vi "Change Tag Name.vi"(6 "Variant":variant, 8 "error in":errorcluster, 9 "old values":string[][](array[string]), 10 "object ref in":T1, 11 "Cluster":T2) -> (0 "error out":errorcluster)   [LabVIEW 2013, in "Shared Memory Editor Node.lvclass"]
doc: "Copyright 2016 National Instruments Corporation\n\nLicensed under the Apache License, Version 2.0 (the \"License\"); you may not use this file except in compliance with the License. You may obtain a copy of the License at http://www.apache.org/licenses/LICENSE-2.0\nUnless required by applicable law or agreed to in writing, software distributed under the License is distributed on an \"AS IS\" BASIS, WITHOUT WARRANTIES OR CONDITIONS OF ANY KIND, either express or implied. See the License for the specific language governing permissions and limitations under the License."
uses:
  Shared Memory Editor Node.lvclass
  <vilib>/NI/DCAF Table API/Table Manager/Cell Change.ctl
  <vilib>/NI/DCAF Table API/Table Manager/object ref.ctl
  <vilib>/NI/DCAF/Tag Editor Core/Configuration Editor/Classes/Engine Parent/Engine Parent Editor Node.lvclass
  <vilib>/NI/DCAF/Tag Editor Core/Configuration Editor/Classes/Module editor node/module editor node.lvclass
  module/configuration/Shared Memory Configuration.lvclass
  module/configuration/Shared Memory Configuration.lvclass/Shared Memory Configuration.ctl
  <vilib>/NI/DCAF Table API/Table Manager.lvlib
  <vilib>/NI/DCAF Table API/Table Manager/Table Manager.lvclass
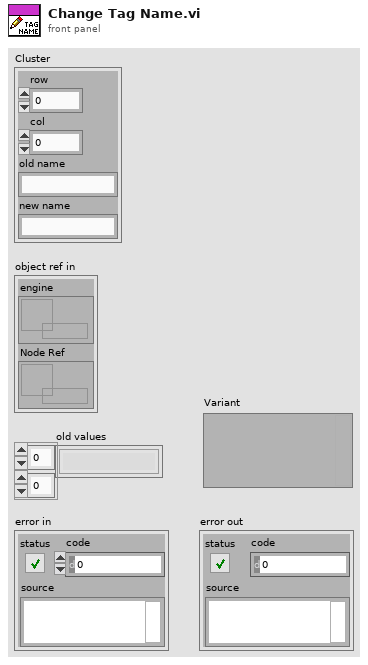
[diagram p1: front panel]
types:
  T1 = typedef "Table Manager.lvlib/Table Manager.lvclass/object ref.ctl" = cluster{"engine":refnum<data-value>, "Node Ref":refnum<data-value>}
  T2 = typedef "Table Manager.lvlib/Cell Change.ctl" = cluster{"row":i32, "col":i32, "old name":string, "new name":string}
  T3 = typedef "Shared Memory Configuration.lvclass/line configuration.ctl" = cluster{"name":string, "data type":T4, "channel":refnum<class "TBM channel.lvclass">}
  T4 = typedef "tag bus.lvlib/tag descriptor.lvclass/Data Type.ctl" = enum16{"Double", "Single", "I64", "I32", "I16", "I8", "U64", "U32", "U16", "U8", "Boolean", "String", "Array of Double", "Array of Single", "Array of I64", "Array of I32", "Array of I16", "Array of I8", "Array of U64", "Array of U32", "Array of U16", "Array of U8", "Array of Boolean", "Array of String"}
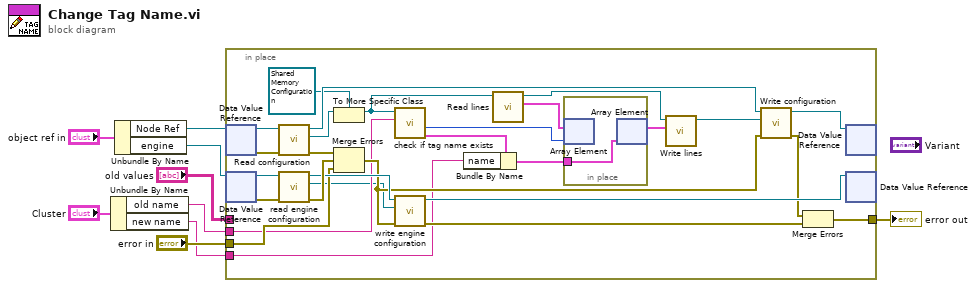
[diagram p0: block diagram]
diagram:
  n1 = Unbundle By Name("Cluster") -> ("old name"=w2:string, "new name"=w1:string)
  n2 = Unbundle By Name("object ref in") -> ("Node Ref"=w4:refnum<data-value>, "engine"=w3:refnum<data-value>)
  n3 = in-place {
    in-place-border: [w29] -> w8
    in-place-border: "error in" -> [w21]
    in-place-border: "old values" -> [_]
    in-place-border: w2 -> [w15]
    in-place-border: w1 -> [w11]
    n4 = in-place-dvr #1(w4) -> (w26:refnum<class "module editor node.lvclass">, w28:errorcluster)
    n5 = in-place-dvr #2(w3) -> (w36:refnum<class "Engine Parent Editor Node.lvclass">, w37:errorcluster)
    n6 = call-dynamic "Read configuration.vi"("error in"=w28, "NISE_CEF_serializable node in"=w26) -> ("error out"=w27:errorcluster, "configuration"=w24:refnum<class "NISE_CEF_serializable configuration.lvclass">, "NISE_CEF_serializable node out"=w25:refnum<class "module editor node.lvclass">)  [unwired: 7 in]
    n7 = call <vilib>:"read engine configuration.vi"("error in"=w37, "Engine Parent Editor Node in"=w36) -> ("error out"=w33:errorcluster, "engine configuration"=w13:refnum<class "engine configuration.lvclass">, "Engine Parent Editor Node out"=w32:refnum<class "Engine Parent Editor Node.lvclass">)  [unwired: 7 in]
    n8 = To More Specific Class(target class=refnum<class "Shared Memory Configuration.lvclass"> refnum ("tag select module configuration"), reference=w24) -> (specific class reference=w20:refnum<class "Shared Memory Configuration.lvclass">)  [unwired: 1 in, 1 out]
    n9 = Merge Errors(w27, w33, w21) -> (w23:errorcluster)
    n10 = call "check if tag name exists.vi"("name to locate"=w15, "shared memory module configuration in"=w20) -> ("tag config"=w16:T3, "index"=w17:i32)  [unwired: 6 in, 2 out]
    n11 = call <vilib>:"write engine configuration.vi"("error in"=w23, "engine configuration"=w13, "Engine Parent Editor Node in"=w32) -> ("error out"=w31:errorcluster, "Engine Parent Editor Node out"=w35:refnum<class "Engine Parent Editor Node.lvclass">)  [unwired: 7 in]
    n12 = Bundle By Name(cluster=w16, "name"=w11) -> (w14:T3)
    n13 = call "Read lines.vi"("shared memory module configuration"=w20) -> ("lines"=w19:T3[], "shared memory module configuration out"=w18:refnum<class "Shared Memory Configuration.lvclass">)  [unwired: 8 in, 1 out]
    n14 = in-place {
      in-place-border: w14 -> [w38]
      n15 = in-place-array #3(w19, w17) -> ()  [unwired: 1 out]
      n16 = in-place-array #3(w38) -> (w12:T3[])  [unwired: 1 out]
    }
    n17 = call "Write lines.vi"("lines"=w12, "shared memory module configuration"=w18) -> ("shared memory module configuration out"=w10:refnum<class "Shared Memory Configuration.lvclass">)  [unwired: 8 in, 1 out]
    n18 = call-dynamic "Write configuration.vi"("error in"=w23, "configuration"=w10, "NISE_CEF_serializable node in"=w25) -> ("error out"=w30:errorcluster, "NISE_CEF_serializable node out"=w34:refnum<class "module editor node.lvclass">)  [unwired: 7 in]
    n19 = Merge Errors(w30, w31) -> (w29:errorcluster)
    n20 = in-place-dvr #1(w34) -> ()  [unwired: 2 out]
    n21 = in-place-dvr #2(w35) -> ()  [unwired: 2 out]
  }
  "error out" <- w8
